vi "Get_Indicies_and_Number_of_Jumps-5.vi"(5 "[IN] Index of connected\ntracks with problem dot":i32[](array[numeric]), 6 "[IN] Index of connected \ndots inside the track":i32[](array[numeric]), 8 "[IN] # of Track with\nFirst Problem Point":i32, 9 "[IN] Index of First Pro\nblem Point Inside Track":i32, 10 "[IN] Still connected\ntracks in group":T1) -> (3 "[OUT] Indicies for Jumps":i32[](array[numeric]))   [LabVIEW 2017]
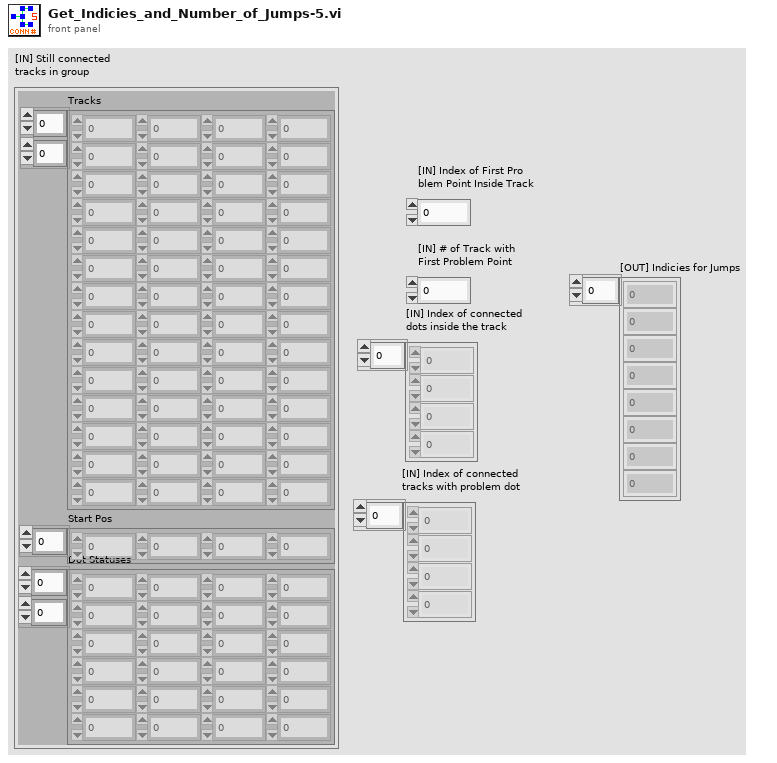
[diagram p1: front panel]
types:
  T1 = cluster{"Tracks":dbl[][], "Start Pos":i32[], "Dot Statuses":i16[][]}
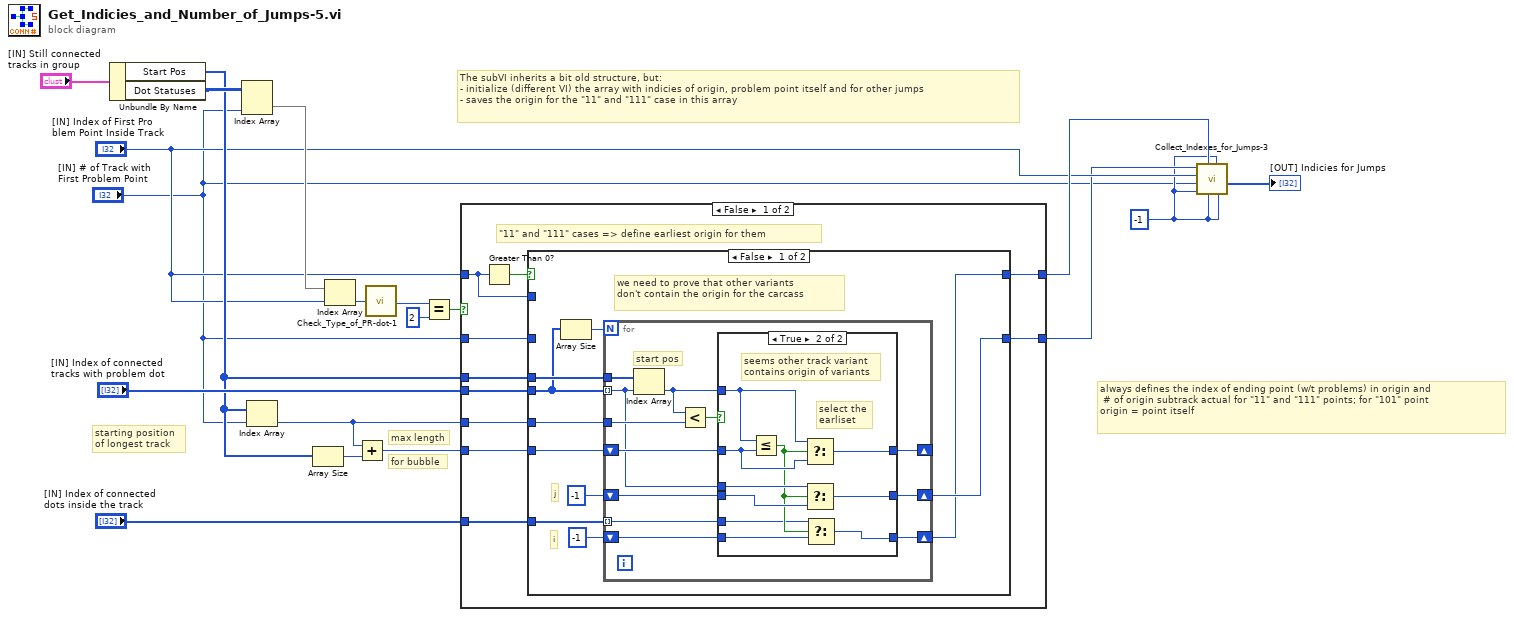
[diagram p0: block diagram]
diagram:
  w2 = -1 ("[IN] # Track with \nSecond Problem Point")
  # "always defines the index of ending point (w/t problems) in origin and\n # of origin subtrack actual for \"11\" and \"111\" points; for \"101\" point \norigin = point itself"
  # "for bubble"
  # "max length"
  # "starting position \nof longest track"
  # "The subVI inherits a bit old structure, but:  \n- initialize (different VI) the array with indicies of origin, problem point itself and for other jumps\n- saves the origin for the \"11\" and \"111\" case in this array"
  n1 = Unbundle By Name("[IN] Still connected\ntracks in group") -> ("Start Pos"=w11:i32[], "Dot Statuses"=w18:i16[][])
  n2 = Index Array(array=w18, index (col)="[IN] # of Track with\nFirst Problem Point") -> (element=w6:i16[])  [unwired: 1 in]
  n3 = Index Array(array=w11, index="[IN] # of Track with\nFirst Problem Point") -> (element=w10:i32)
  n4 = Array Size(array=w11) -> (size(s)=w9:i32)
  n5 = Index Array(array=w6, index="[IN] Index of First Pro\nblem Point Inside Track") -> (element=w17:i16)
  n6 = Add(x=w10, y=w9) -> (x+y=w8:i32)
  n7 = call "Check_Type_of_PR-dot-1.vi"("[IN] dot status"=w17) -> ("[OUT] Type of\nproblem dot"=w16:i32)
  n8 = Equal?(x=w16, y=2) -> (x = y?=w14:bool)
  n9 = case shown="False" w14 {
    tunnel: [w27 w67] -> w5
    tunnel: "[IN] Index of First Pro\nblem Point Inside Track" -> [w28 w67]
    tunnel: [w25 w68] -> w3
    tunnel: "[IN] # of Track with\nFirst Problem Point" -> [w26 w68]
    tunnel: "[IN] Index of connected\ntracks with problem dot" -> [w24 _]
    tunnel: w10 -> [w23 _]
    tunnel: w11 -> [w22 _]
    tunnel: w8 -> [w21 _]
    tunnel: "[IN] Index of connected \ndots inside the track" -> [w20 _]
    frame False {
      # "\"11\" and \"111\" cases => define earliest origin for them"
      n10 = Greater Than 0?(x=w28) -> (x > 0?=w29:bool)
      n11 = case shown="False" w29 {
        tunnel: w28 -> [_ w65]
        tunnel: [w30 w65] -> w27
        tunnel: w26 -> [_ w66]
        tunnel: [w33 w66] -> w25
        tunnel: w24 -> [w36 _]
        tunnel: w23 -> [w38 _]
        tunnel: w22 -> [w37 _]
        tunnel: w21 -> [w35 _]
        tunnel: w20 -> [w31 _]
        frame False {
          # "i"
          # "j"
          # "we need to prove that other variants\ndon't contain the origin for the carcass"
          n12 = Array Size(array=w36) -> (size(s)=w39:i32)
          n13 = for {
            N: w39 -> [_]
            tunnel: w36 -> [w43] mode=indexing
            tunnel: w38 -> [w50]
            tunnel: w37 -> [w51]
            shift-right: [w47] -> _
            shift-left: w35 -> [w48]
            shift-right: [w44] -> w33
            shift-left: -1 -> [w45]
            shift-right: [w40] -> w30
            shift-left: -1 -> [w42]
            tunnel: w31 -> [w41] mode=indexing
            # "start pos"
            n14 = Index Array(array=w51, index=w43) -> (element=w46:i32)
            n15 = Less?(x=w46, y=w50) -> (x < y?=w49:bool)
            n16 = case shown="True" w49 {
              tunnel: w48 -> [w54 w62]
              tunnel: [w54 w64] -> w47
              tunnel: w46 -> [_ w63]
              tunnel: w45 -> [w53 w60]
              tunnel: [w53 w59] -> w44
              tunnel: w43 -> [_ w61]
              tunnel: w42 -> [w52 w56]
              tunnel: w41 -> [_ w57]
              tunnel: [w52 w55] -> w40
              frame False {
              }
              frame True {
                # "select the \nearliset"
                # "seems other track variant\ncontains origin of variants"
                n17 = Less Or Equal?(x=w63, y=w62) -> (x <= y?=w58:bool)
                n18 = Select(t=w63, s=w58, f=w62) -> (s? t:f=w64:i32)
                n19 = Select(t=w61, s=w58, f=w60) -> (s? t:f=w59:i32)
                n20 = Select(t=w57, s=w58, f=w56) -> (s? t:f=w55:i32)
              }
            }
          }
        }
        frame True {
          # "so this subtrack already contains the origin"
        }
      }
    }
    frame True {
    }
  }
  n21 = call "Collect_Indexes_for_Jumps-3.vi"("[IN] # Track with \nThird Problem Point"=w2, "[IN] Index of Third\nProblem point"=w2, "[IN] # Track with \nSecond Problem Point"=w2, "[IN] Index of Point Be\nfore Problem (Origin)"=w5, "[IN] Index of Second\nProblem point"=w2, "[IN] # Track with First\nProblem Point"="[IN] # of Track with\nFirst Problem Point", "[IN] Index of First \nProblem Point"="[IN] Index of First Pro\nblem Point Inside Track", "[IN] # Track of Origin"=w3) -> ("[OUT] Indexes for Jumps"=→"[OUT] Indicies for Jumps":i32[])  [unwired: 3 in]
